vi "meds_escala.vi"(2 "F. Escala":u8, 3 "linealidad":u8, 4 "Med IN":i16) -> (0 "Med OUT num":dbl, 1 "F. Escala out":dbl)   [LabVIEW 2010]
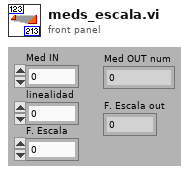
[diagram p1: front panel]
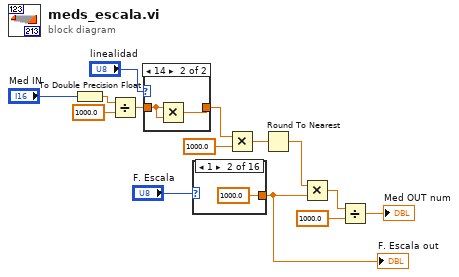
[diagram p0: block diagram]
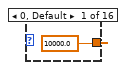
[diagram p2: hidden frame]
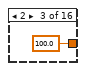
[diagram p3: hidden frame]
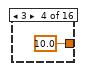
[diagram p4: hidden frame]
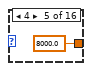
[diagram p5: hidden frame]
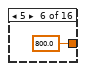
[diagram p6: hidden frame]
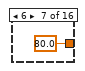
[diagram p7: hidden frame]
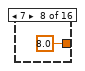
[diagram p8: hidden frame]
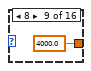
[diagram p9: hidden frame]
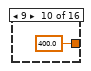
[diagram p10: hidden frame]
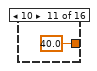
[diagram p11: hidden frame]
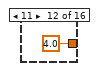
[diagram p12: hidden frame]
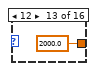
[diagram p13: hidden frame]
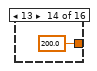
[diagram p14: hidden frame]
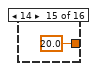
[diagram p15: hidden frame]
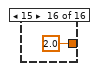
[diagram p16: hidden frame]
diagram:
  n1 = To Double Precision Float(number="Med IN") -> (double precision float=w2:dbl)
  n2 = Divide(x=w2, y=1000.0) -> (x/y=w13:dbl)
  n3 = case shown="14" "linealidad" {
    tunnel: [w15 w17] -> w6
    tunnel: w13 -> [w15 w16]
    frame 15, Default {
    }
    frame 14 {
      n4 = Multiply(x=w16, y=w16) -> (x*y=w17:dbl)
    }
  }
  n5 = case shown="1" "F. Escala" {
    tunnel: [10000.0 ("y") 1000.0 ("y") 100.0 ("y") 10.0 ("y") 8000.0 ("y") 800.0 ("y") 80.0 ("y") 8.0 ("y") 4000.0 ("y") 400.0 ("y") 40.0 ("y") 4.0 ("y") 2000.0 ("y") 200.0 ("y") 20.0 ("y") 2.0 ("y")] -> w9
    frame 0, Default {
    }
    frame 1 {
    }
    frame 2 {
    }
    frame 3 {
    }
    frame 4 {
    }
    frame 5 {
    }
    frame 6 {
    }
    frame 7 {
    }
    frame 8 {
    }
    frame 9 {
    }
    frame 10 {
    }
    frame 11 {
    }
    frame 12 {
    }
    frame 13 {
    }
    frame 14 {
    }
    frame 15 {
    }
  }
  "F. Escala out" <- w9
  n6 = Multiply(x=w6, y=1000.0) -> (x*y=w4:dbl)
  n7 = Round To Nearest(number=w4) -> (nearest integer value=w3:dbl)
  n8 = Multiply(x=w3, y=w9) -> (x*y=w5:dbl)
  n9 = Divide(x=w5, y=1000.0) -> (x/y=→"Med OUT num":dbl)
